vi "RecordLatch.vi"(7 "Rec Button":bool) -> (2 "Indicator":bool, 3 "Record":bool)   [LabVIEW 2016]
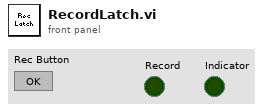
[diagram p1: front panel]
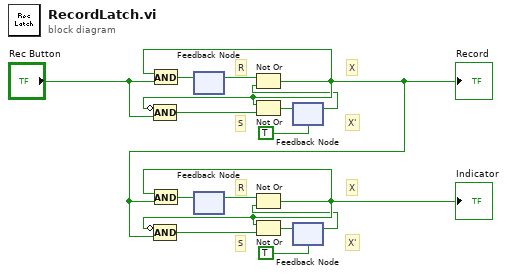
[diagram p0: block diagram]
diagram:
  # "X'"
  # "X"
  # "S"
  # "R"
  # "X'"
  # "X"
  # "S"
  # "R"
  n1 = feedback #1() -> (w5:bool)  [unwired: 1 in]
  n2 = feedback #2() -> (w12:bool)  [unwired: 1 in]
  n3 = feedback #3(TRUE) -> (w2:bool)
  n4 = Not Or(1:w2, 2:w5) -> (0:w14:bool)
  "Record" <- w14
  n5 = And(x=w14, y="Rec Button") -> (x .and. y?=w4:bool)
  n6 = Compound Arithmetic op=AND(invert w14, "Rec Button") -> (w6:bool)
  n7 = feedback-in #1(w4) -> ()
  n8 = Not Or(1:w6, 2:w14) -> (0:w1:bool)
  n9 = feedback-in #3(w1) -> ()
  n10 = feedback #4(TRUE) -> (w9:bool)
  n11 = Not Or(1:w9, 2:w12) -> (0:w15:bool)
  "Indicator" <- w15
  n12 = And(x=w15, y=w14) -> (x .and. y?=w11:bool)
  n13 = Compound Arithmetic op=AND(invert w15, w14) -> (w13:bool)
  n14 = feedback-in #2(w11) -> ()
  n15 = Not Or(1:w13, 2:w15) -> (0:w8:bool)
  n16 = feedback-in #4(w8) -> ()
